vi "LVClass_Camera SnapImage.vi"(0 "Camera in":refnum<class "Camera.lvclass">, 5 "Image":refnum<class "Image.lvclass">, 7 "Image RAW":refnum<class "Image.lvclass">, 9 "remove_background":bool=TRUE, 11 "error in (no error)":errorcluster) -> (4 "Camera out":refnum<class "Camera.lvclass">, 6 "Image (dup)":refnum<class "Image.lvclass">, 8 "Image (dup) RAW":refnum<class "Image.lvclass">, 15 "error out":errorcluster)   [LabVIEW 2020, in "Camera.lvclass"]
doc: "Snap Image using new acquisition mode and synchronous synchronization mode.\nThere is no need of Starting and Stopping the camera manually with this\nmethod.\n\n<B>CameraIn</B> : Camera object.\n<B>CameraOut</B> : Camera object.\n<B>Image</B> : Captured image with (optionnally) background removed.\n<B>remove_background</B> : Boolean which indicates if background should be substracted.\n<B>RawImage</B> : Captured image without any post-processing applied."
uses:
  Camera.lvclass
  Image.lvclass
  Camera.lvclass/Camera.ctl
  LVClass_Image read Image Compat ptr.vi
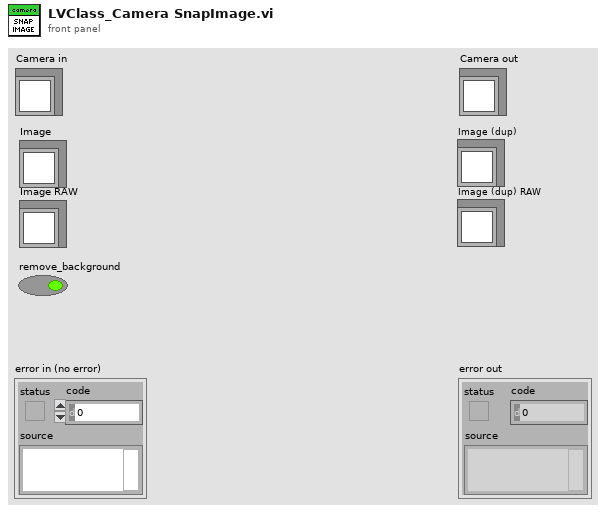
[diagram p1: front panel]
types:
  T1 = typedef "ClassID.ctl" = i64
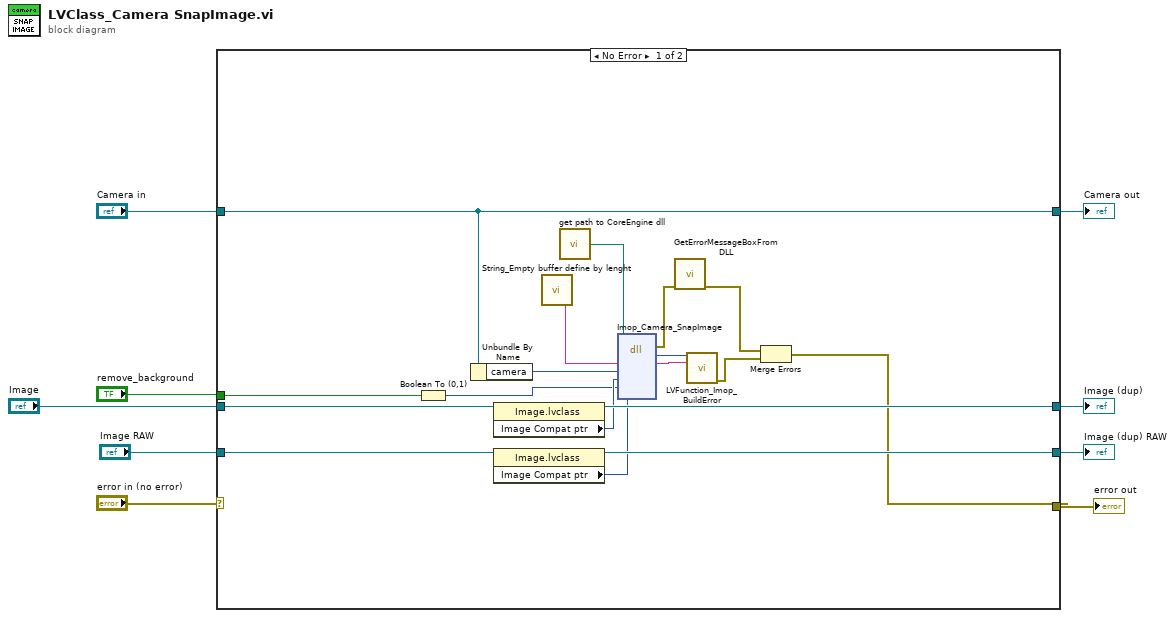
[diagram p0: block diagram]
diagram:
  n1 = case shown="No Error" "error in (no error)" {
    selector: "error in (no error)" -> [_ w31]
    tunnel: [w22 w31] -> w8
    tunnel: [w21 w30] -> w6
    tunnel: "Camera in" -> [w21 w30]
    tunnel: [w26 w29] -> w5
    tunnel: "Image" -> [w27 w29]
    tunnel: "Image RAW" -> [w25 w28]
    tunnel: [w24 w28] -> w2
    tunnel: "remove_background" -> [w23 _]
    frame No Error {
      n2 = Boolean To (0,1)(Boolean=w23) -> (0, 1=w12:i16)
      n3 = Unbundle By Name(w21) -> ("camera"=w17:T1)
      n4 = property class="Image.lvclass"(reference=w27) -> (reference out=w26:refnum<class "Image.lvclass">, "Image Compat ptr"=w15:T1)  [unwired: 1 in, 1 out]
      n5 = property class="Image.lvclass"(reference=w25) -> (reference out=w24:refnum<class "Image.lvclass">, "Image Compat ptr"=w13:T1)  [unwired: 1 in, 1 out]
      n6 = call "String_Empty buffer define by lenght.vi"() -> ("Empty buffer"=w20:string)  [unwired: 1 in]
      n7 = call "get path to CoreEngine dll.vi"() -> ("path to wavekit library"=w16:path)  [unwired: 14 in, 1 out]
      n8 = dll-call lib="D:/FLE/0.Code/CoreEngine4_Suite_v4.1/LV2011_interface/DLLs/c_interface_vc100.dll" fn="Imop_Camera_SnapImage"(path in=w16, "message"=w20, "camera"=w17, "HASO_image"=w15, "remove background"=w12, "RAW HASO_image"=w13) -> (error out=w14:errorcluster, "return type"=w19:i32, "message"=w18:string)  [unwired: 6 in, 1 out]
      n9 = call "GetErrorMessageBoxFromDLL.vi"("error IN"=w14) -> ("error OUT"=w11:errorcluster)  [unwired: 10 in]
      n10 = call "LVFunction_Imop_BuildError.vi"("code"=w19, "String to Prepend to source (\"\")"=w18) -> ("error out"=w10:errorcluster)  [unwired: 13 in]
      n11 = Merge Errors(w11, w10) -> (w22:errorcluster)
    }
    frame Error {
    }
  }
  "error out" <- w8
  "Camera out" <- w6
  "Image (dup)" <- w5
  "Image (dup) RAW" <- w2
